vi "digWaveFromPlatData_Automatic.vi"(6 "mazeDirection":string, 8 "error in (no error)":errorcluster, 9 "Platforms\nto lower":i32[](array[numeric]), 11 "Platforms\nto raise":i32[](array[numeric])) -> (0 "error out":errorcluster)   [LabVIEW 2017]
uses:
  <vilib>/Utility/error.llb/DialogType.ctl
  <vilib>/imath/engines/lvmath2/RunTimeEngine/BuiltInFunctions/length/NIMS_length(GV).vi
  <instcachedir>/0/NIMS_length(GV)_08A3D13377FD4E4B96F5795FBF3698FA.lvgen/NIMS_length(GV)_08A3D13377FD4E4B96F5795FBF3698FA_003.vi
  <vilib>/imath/engines/lvmath2/RunTimeEngine/BuiltInFunctions/repeatmx/NIMS_repeatmx(GM, I32, I32).vi
  <instcachedir>/0/NIMS_repeatmx(GM, I32, I32)_8EDBB852F26742A48D04758F158AC943.lvgen/NIMS_repeatmx(GM, I32, I32)_8EDBB852F26742A48D04758F158AC943_004.vi
  <vilib>/imath/engines/lvmath2/RunTimeEngine/RowToken/NIMS_RowToken_SorRV_M.vi
  <instcachedir>/0/NIMS_RowToken_SorRV_M_997882E9B890466D9AE38E5C4E8B9D70.lvgen/NIMS_RowToken_SorRV_M_997882E9B890466D9AE38E5C4E8B9D70_000.vi
  <vilib>/imath/engines/lvmath2/RunTimeEngine/ErrorHandling/NIMS_Create Error From Enums.vi
  <vilib>/imath/engines/lvmath2/RunTimeEngine/BuiltInFunctions/mirrorh/NIMS_mirrorh(GRowV).vi
  <instcachedir>/0/NIMS_mirrorh(GRowV)_B6A8CC4EAFBA4F9A82A59460D67BDFF0.lvgen/NIMS_mirrorh(GRowV)_B6A8CC4EAFBA4F9A82A59460D67BDFF0_000.vi
  <vilib>/imath/engines/lvmath2/RunTimeEngine/MatrixToken/NIMS_MatrixToken_RV_RV.vi
  <instcachedir>/0/NIMS_MatrixToken_RV_RV_8B087EE0EE16477EBE1C341EABB504F3.lvgen/NIMS_MatrixToken_RV_RV_8B087EE0EE16477EBE1C341EABB504F3_002.vi
  <vilib>/imathl/engines/lvmath/Functions/Error Handling/Create Error.vi
  <vilib>/imath/engines/lvmath2/RunTimeEngine/IndexRead/NIMS M($).vi
  <instcachedir>/0/NIMS M($)_82D1177398184AFB96A6AFB63C3C3F57.lvgen/NIMS M($)_82D1177398184AFB96A6AFB63C3C3F57_005.vi
  <vilib>/imath/engines/lvmath2/RunTimeEngine/MatrixToken/NIMS_MatrixToken_M_RV.vi
  <instcachedir>/0/NIMS_MatrixToken_M_RV_EE6E048DE0454E429C3E3ED099F2A9DF.lvgen/NIMS_MatrixToken_M_RV_EE6E048DE0454E429C3E3ED099F2A9DF_002.vi
  <vilib>/imath/engines/lvmath2/RunTimeEngine/NodeEndStatement/NIMS_NodeEndStatement_Output.vi
  <instcachedir>/0/NIMS_NodeEndStatement_Output_53EC0D466D134D7ABD903AC30B43404B.lvgen/NIMS_NodeEndStatement_Output_53EC0D466D134D7ABD903AC30B43404B_012.vi
  <vilib>/imath/engines/lvmath2/RunTimeEngine/ErrorHandling/NIMS_Finalize Error.vi
panel:
  out "message":string=" INSTRUCTIONS:\r\rNormal Use:  When using subVIs that incorporate the error in/error out (or error I/O) structure, place this handler where you want to inform the user of an error, typically at the end of the I/O data path, as the last action of the program.  If the error in error? is ERROR, the handler creates a message describing the error and its source.  If the type of dialog = 1 (default), the message is displayed to the user, who can only acknowedge it.  If the type = 2, the user can acknowledge the message or abort execution; aborting a program with active I/O is not recommended.  If the type = 0, no message is displayed; this is used to process the error programmatically, and the error out cluster elements are wired to individual terminals for that reason.  \r\rOther Use:\n\r\nlocal testing.  To test the error code of a subVI or function that does not have the error I/O structure, you can wire its error code and a source string to the local error code and error source inputs.  If error in error? indicates no error and error code is not equal to 0, the local code and source are substituted for the error in values, and error? is set TRUE (ERROR)."
  out "source out":string
  out "code out":i32 format="%0.0f"
  out "error?":bool
  in  "type of dialog (OK msg:1)":T1=1 items=["no dialog", "OK message", "continue or stop message", "OK message + warnings", "continue/stop + warnings"]
  in  "error source (\" \")":string
  in  "error code (no error:0)":i32 format="%0.0f"
  out "Digital Waveform Graph 3":digitalwaveform(graph)
  out "Digital Waveform Graph":digitalwaveform(graph)
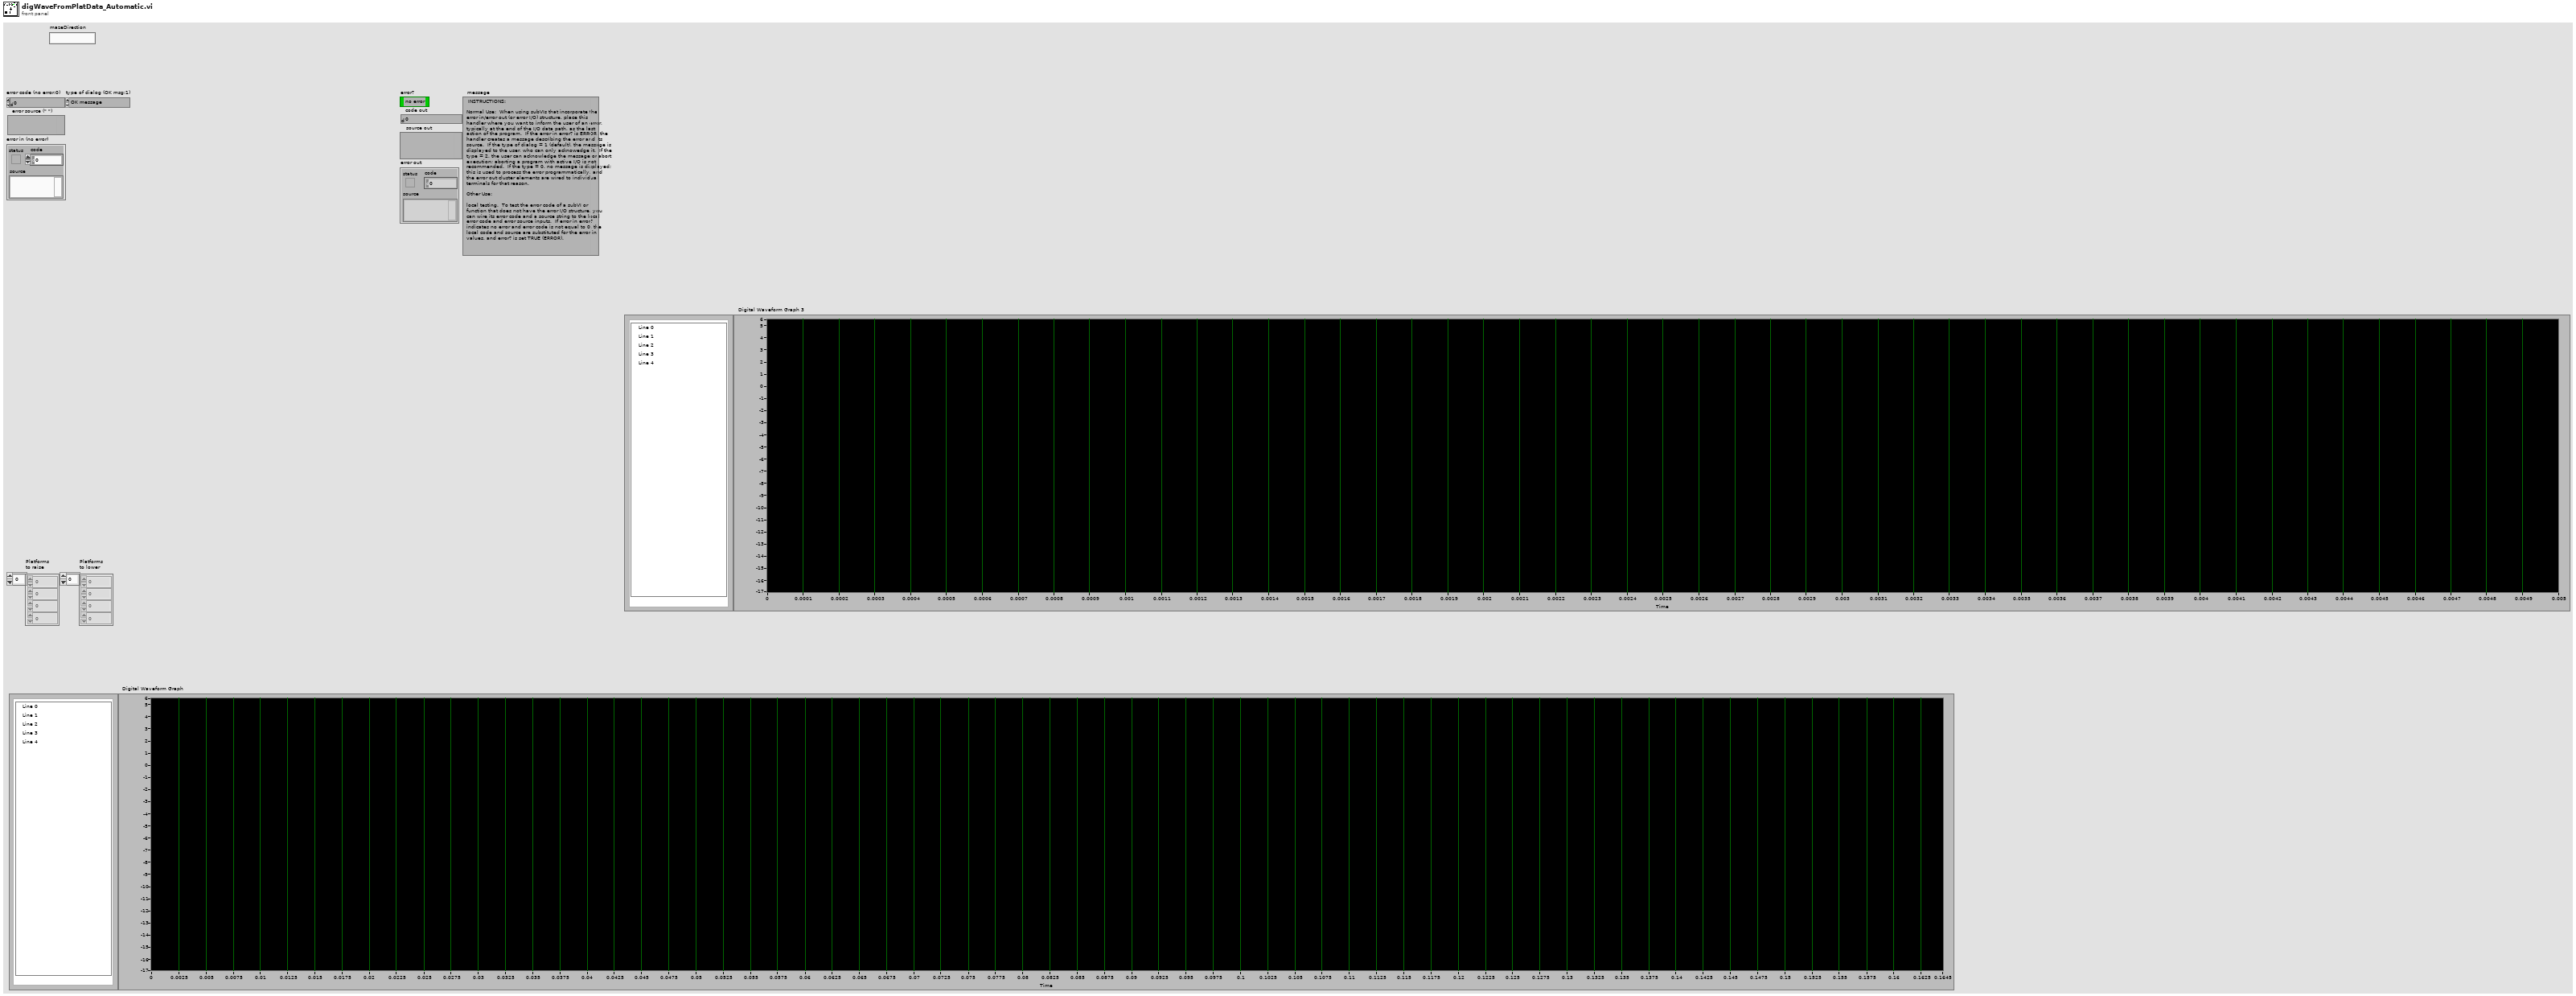
[diagram p1: front panel]
types:
  T1 = typedef "DialogType.ctl" = u16
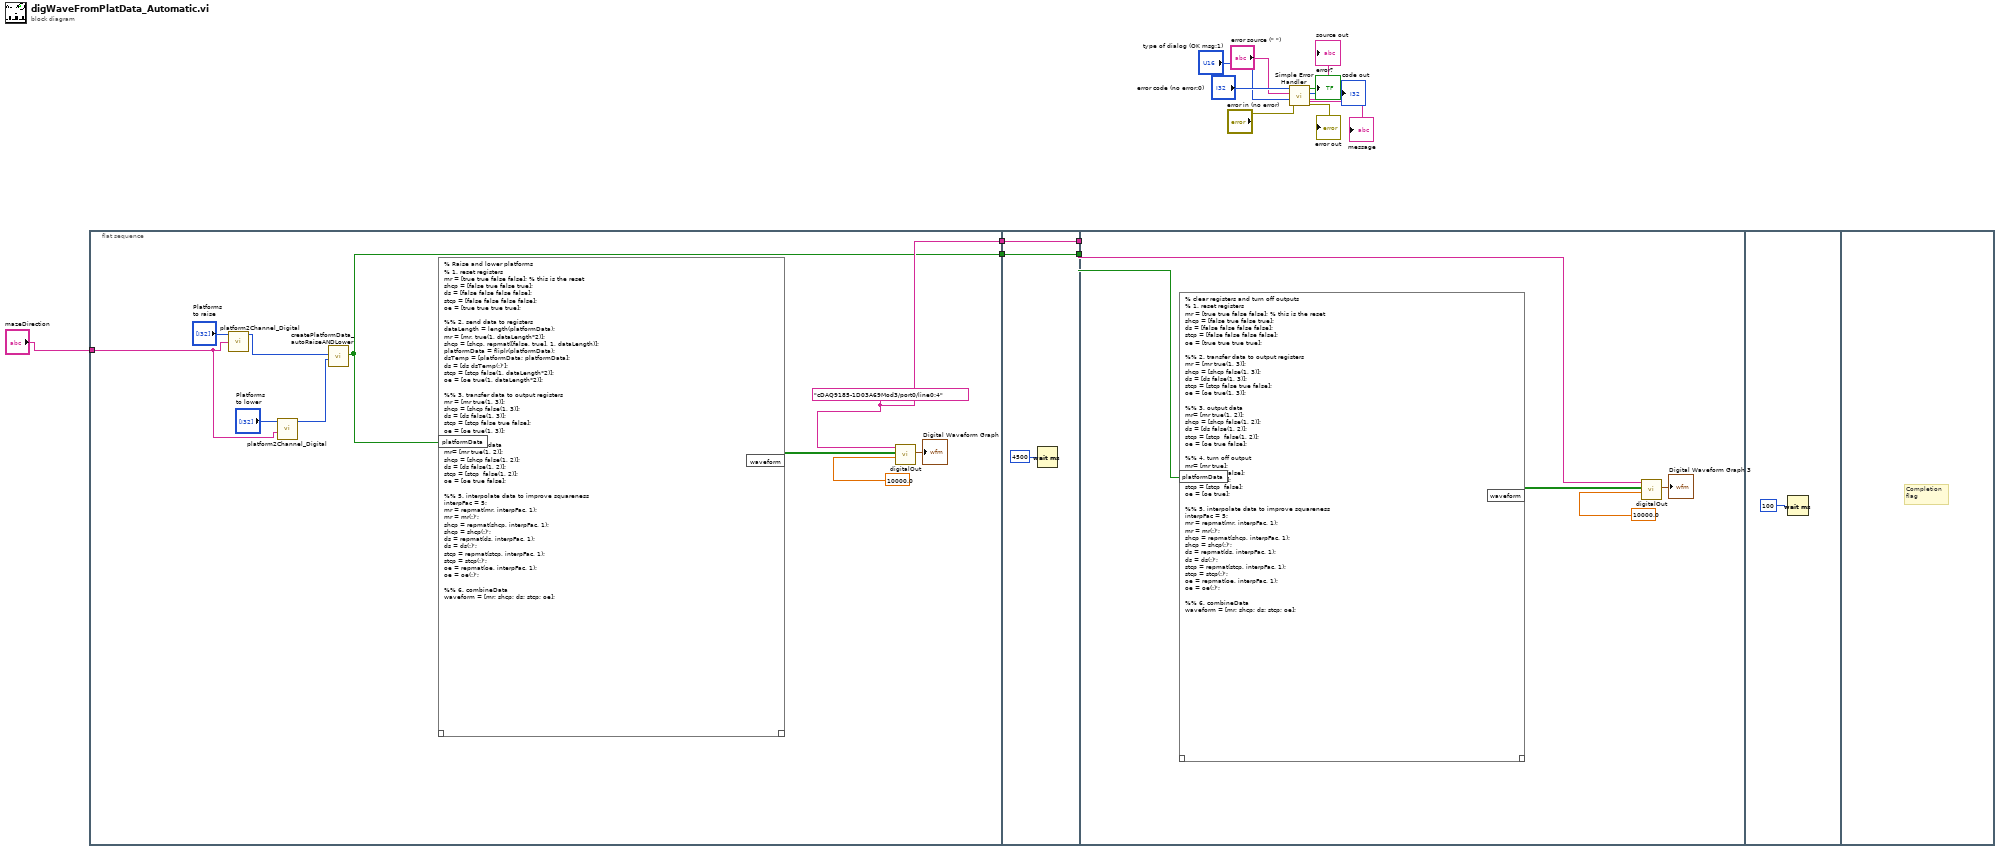
[diagram p0: block diagram]
diagram:
  n1 = flat-sequence {
    tunnel: [w20] -> w14
    tunnel: [w21] -> w13
    tunnel: "mazeDirection" -> [w15]
    tunnel: w14 -> [w498]
    tunnel: [w498] -> w12
    tunnel: w13 -> [w497]
    tunnel: [w497] -> w11
    tunnel: w12 -> [w504]
    tunnel: w11 -> [w500]
    frame #0 {
      w21 = tag "cDAQ9185-1D03A69Mod3/port0/line0:4" ("lines")
      n2 = call "platform2Channel_Digital.vi"("mazeDirection"=w15, "Platforms"="Platforms\nto raise") -> ("channels"=w19:i32[])  [unwired: 9 in]
      n3 = call "platform2Channel_Digital.vi"("mazeDirection"=w15, "Platforms"="Platforms\nto lower") -> ("channels"=w18:i32[])  [unwired: 9 in]
      n4 = call "createPlatformData_autoRaiseANDLower.vi"("Plaforms to raise"=w19, "Plaforms to lower"=w18) -> ("platformData"=w20:bool[])  [unwired: 8 in]
      n5 = mathscript code="% Raise and lower platforms\n% 1. reset registers\nmr = [true true false false]; % this is the reset\nshcp = [false true false true];\nds = [false false false false];\nstcp = [false false false false];\noe = [true true true true];\n\n%% 2. send data to registers\ndataLength = length(platformData); \nmr = [mr, true(1, dataLength*2)];\nshcp = [shcp, repmat([false, true], 1, dataLength)];\nplatformData = fliplr(platformData);\ndsTemp = [platformData; platformData];\nds = [ds dsTemp(:)'];\nstcp = [stcp false(1, dataLength*2)];\noe = [oe true(1, dataLength*2)];\n\n%% 3. transfer data to output registers\nmr = [mr true(1, 3)];\nshcp = [shcp false(1, 3)];\nds = [ds false(1, 3)];\nstcp = [stcp false true false];\noe = [oe true(1, 3)];\n\n%% 4. output data\nmr= [mr true(1, 2)];\nshcp = [shcp false(1, 2)];\nds = [ds false(1, 2)];\nstcp = [stcp  false(1, 2)];\noe = [oe true false];\n\n%% 5. interpolate data to improve squareness\ninterpFac = 5;\nmr = repmat(mr, interpFac, 1);\nmr = mr(:)';\nshcp = repmat(shcp, interpFac, 1);\nshcp = shcp(:)';\nds = repmat(ds, interpFac, 1);\nds = ds(:)';\nstcp = repmat(stcp, interpFac, 1);\nstcp = stcp(:)';\noe = repmat(oe, interpFac, 1);\noe = oe(:)';\n\n%% 6. combineData\nwaveform = [mr; shcp; ds; stcp; oe];"("platformData"=w20) -> ("waveform"=w23:bool[][])  [unwired: 1 in, 1 out]
      n6 = call "digitalOut.vi"("rate"=10000.0, "waveform"=w23, "lines"=w21) -> ("digital waveform"=→"Digital Waveform Graph":digitalwaveform)  [unwired: 8 in]
    }
    frame #1 {
      n7 = Wait (ms)(milliseconds to wait=4500) -> ()  [unwired: 1 out]
    }
    frame #2 {
      n8 = mathscript code="% clear registers and turn off outputs\n% 1. reset registers\nmr = [true true false false]; % this is the reset\nshcp = [false true false true];\nds = [false false false false];\nstcp = [false false false false];\noe = [true true true true];\n\n%% 2. transfer data to output registers\nmr = [mr true(1, 3)];\nshcp = [shcp false(1, 3)];\nds = [ds false(1, 3)];\nstcp = [stcp false true false];\noe = [oe true(1, 3)];\n\n%% 3. output data \nmr= [mr true(1, 2)];\nshcp = [shcp false(1, 2)];\nds = [ds false(1, 2)];\nstcp = [stcp  false(1, 2)];\noe = [oe true false];\n\n%% 4. turn off output\nmr= [mr true];\nshcp = [shcp false];\nds = [ds false];\nstcp = [stcp  false];\noe = [oe true];\n\n%% 5. interpolate data to improve squareness\ninterpFac = 5;\nmr = repmat(mr, interpFac, 1);\nmr = mr(:)';\nshcp = repmat(shcp, interpFac, 1);\nshcp = shcp(:)';\nds = repmat(ds, interpFac, 1);\nds = ds(:)';\nstcp = repmat(stcp, interpFac, 1);\nstcp = stcp(:)';\noe = repmat(oe, interpFac, 1);\noe = oe(:)';\n\n%% 6. combineData\nwaveform = [mr; shcp; ds; stcp; oe];"("platformData"=w504) -> ("waveform"=w502:bool[][])  [unwired: 1 in, 1 out]
      n9 = call "digitalOut.vi"("rate"=10000.0, "waveform"=w502, "lines"=w500) -> ("digital waveform"=→"Digital Waveform Graph 3":digitalwaveform)  [unwired: 8 in]
    }
    frame #3 {
      n10 = Wait (ms)(milliseconds to wait=100) -> ()  [unwired: 1 out]
    }
    frame #4 {
      # "Completion\nflag"
    }
  }
  n11 = call <vilib>:"Simple Error Handler.vi"("error code (no error:0)"="error code (no error:0)", "error source (\" \")"="error source (\" \")", "type of dialog (OK msg:1)"="type of dialog (OK msg:1)", "error in (no error)"="error in (no error)") -> ("error?"=→"error?":bool, "code out"=→"code out":i32, "source out"=→"source out":string, "error out"=→"error out":errorcluster, "message"=→"message":string)  [unwired: 1 in]
